vi "Convert Turbine RPMs.vi"(11 "RPMs input":i64[](array[numeric])) -> (3 "RPMs Output":i64[](array[numeric]))   [LabVIEW 2024, in "UI.lvlib"]
uses:
  UI.lvlib
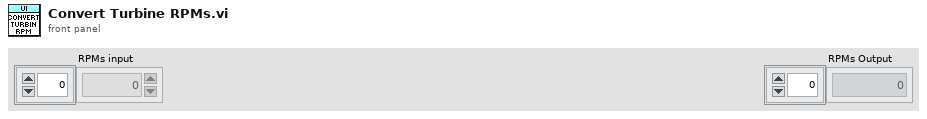
[diagram p1: front panel]
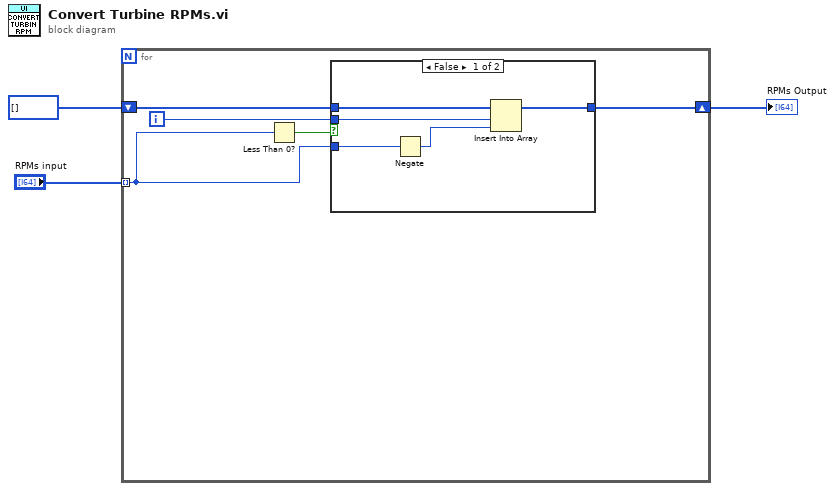
[diagram p0: block diagram]
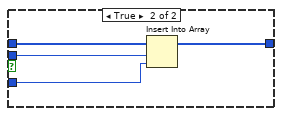
[diagram p2: hidden frame]
diagram:
  n1 = for {
    shift-right: [w7] -> w2
    shift-left: i64[] [] ("RPMs Output") -> [w8]
    tunnel: "RPMs input" -> [w5] mode=indexing
    i -> [w6]
    n2 = Less Than 0?(x=w5) -> (x < 0?=w4:bool)
    n3 = case shown="False" w4 {
      tunnel: w8 -> [w12 w17]
      tunnel: [w13 w16] -> w7
      tunnel: w6 -> [w11 w15]
      tunnel: w5 -> [w10 w14]
      frame False {
        n4 = Negate(x=w10) -> (-x=w9:i64)
        n5 = Insert Into Array(array=w12, index=w11, new element=w9) -> (w13:i64[])
      }
      frame True {
        n6 = Insert Into Array(array=w17, index=w15, new element=w14) -> (w16:i64[])
      }
    }
  }
  "RPMs Output" <- w2
